vi "buildRampDownWaveform.vi"(4 "Fs":dbl=10000.0, 6 "square wave duty cycle (%)":dbl=20.0 format="%0.2f", 7 "signal type":T1(ring)=enum."Square Wave", 8 "input cluster":cluster{"Fs":dbl, "#s":dbl}={"Fs"=1000.0, "#s"=1000.0}, 9 "amplitude":dbl=2.5, 10 "freq":dbl=40.0, 11 "sec rampdown":dbl=0.5 format="%#_13g") -> (3 "rampDown out":waveform(dbl)={"t0"=timestamp(0 s since 1904-01-01), "dt"=1.0, "Y"=array[62500 elements]})   [LabVIEW 2018]
uses:
  <vilib>/Waveform/WDTOps.llb/WDT Append Waveforms DBL.vi
  <vilib>/measure/NI_MABase.lvlib
panel:
  out "output cluster":cluster{"Fs":dbl, "#s":dbl}
  out "N":i32
  out "Waveform Graph":waveform(dbl)(graph) caption="Optostim waveform"
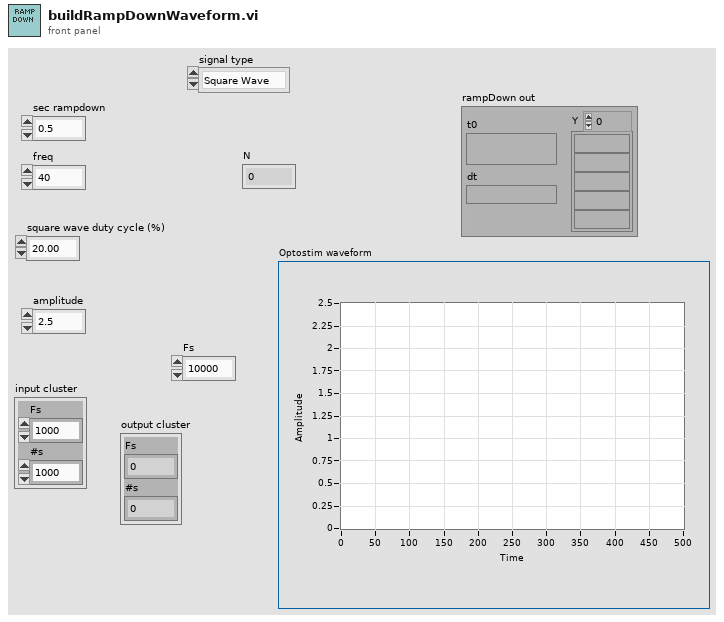
[diagram p1: front panel]
types:
  T1 = enum16{"Sine Wave", "Triangle Wave", "Square Wave", "Sawtooth Wave"}
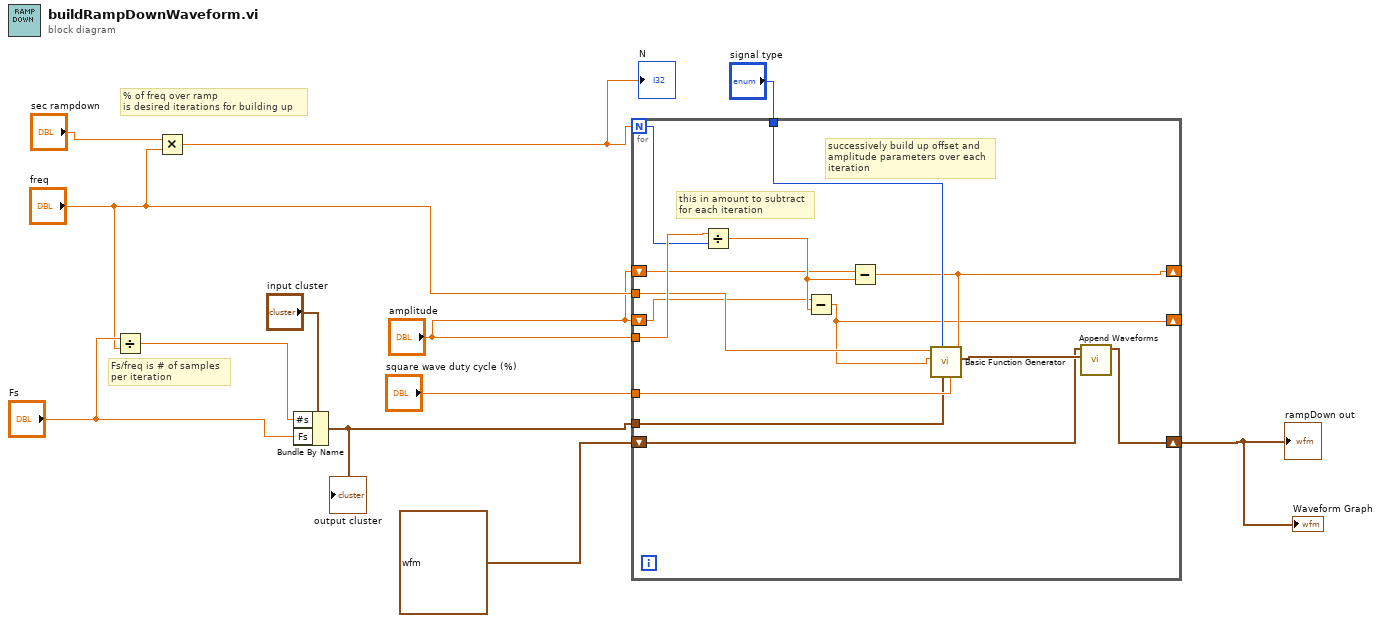
[diagram p0: block diagram]
diagram:
  # "% of freq over ramp\nis desired iterations for building up"
  # "Fs/freq is # of samples \nper iteration"
  n1 = Divide(x="Fs", y="freq") -> (x/y=w8:dbl)
  n2 = Multiply(x="sec rampdown", y="freq") -> (x*y=w2:dbl)
  "N" <- w2
  n3 = Bundle By Name(cluster="input cluster", "#s"=w8, "Fs"="Fs") -> (w7:cluster{"Fs":dbl, "#s":dbl})
  "output cluster" <- w7
  n4 = for {
    N: w2 -> [w21]
    shift-right: [w23] -> w4
    shift-left: waveform(dbl) {"t0"=timestamp(0 s since 1904-01-01), "dt"=1.0, "Y"=[]} ("signal out") -> [w24]
    tunnel: "amplitude" -> [w22]
    shift-right: [w16] -> _
    shift-left: "amplitude" -> [w17]
    tunnel: "signal type" -> [w20]
    tunnel: "freq" -> [w19]
    tunnel: "square wave duty cycle (%)" -> [w18]
    shift-right: [w15] -> _
    shift-left: "amplitude" -> [w13]
    tunnel: w7 -> [w14]
    # "this in amount to subtract\nfor each iteration"
    # "successively build up offset and \namplitude parameters over each\niteration"
    n5 = Divide(x=w22, y=w21) -> (x/y=w26:dbl)
    n6 = Subtract(x=w13, y=w26) -> (x-y=w15:dbl)
    n7 = Subtract(x=w17, y=w26) -> (x-y=w16:dbl)
    n8 = call <vilib>:"Basic Function Generator.vi"("offset"=w16, "square wave duty cycle (%)"=w18, "sampling info"=w14, "signal type"=w20, "amplitude"=w15, "frequency"=w19) -> ("signal out"=w25:waveform(dbl))  [unwired: 3 in, 2 out]
    n9 = call-poly <vilib>:"Append Waveforms.vi"("waveform B"=w25, "waveform A"=w24) -> ("waveform out"=w23:waveform(dbl))  [unwired: 8 in, 1 out]
  }
  "rampDown out" <- w4
  "Waveform Graph" <- w4
